vi "Constructor.vi"(11 "Espresso in":refnum<class "Espresso.lvclass">) -> (3 "Espresso out":refnum<class "Espresso.lvclass">)   [LabVIEW 2013]
uses:
  Espresso.lvclass
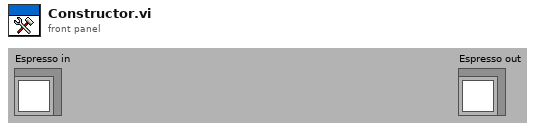
[diagram p1: front panel]
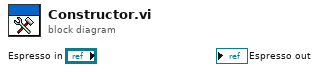
[diagram p0: block diagram]
diagram:
